vi "ButtonReleaseOnClick.vi"(1 "Input":bool) -> (0 "Output":bool)   [LabVIEW 2017]
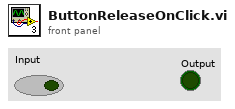
[diagram p1: front panel]
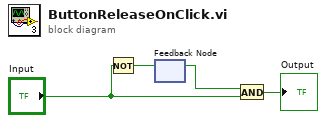
[diagram p0: block diagram]
diagram:
  n1 = Not(x="Input") -> (.not. x?=w4:bool)
  n2 = feedback-in #1(w4) -> ()
  n3 = feedback #1() -> (w3:bool)  [unwired: 1 in]
  n4 = And(x=w3, y="Input") -> (x .and. y?=→"Output":bool)
